vi "Multi-Carrier Modulation Non-Reentrant.vi"(7 "QAM Comparison":enum16{"MT Modulate", "Homebrew"}(ring), 8 "DataLen":i32=512, 9 "QAM Complexity":T1(ring), 10 "Number of Subcarriers":i32, 11 "Lowest f":dbl=1.0 format="%0.2p") -> (0 "FFT Complex":cluster{"f0":dbl, "df":dbl, "real part":dbl[]}(graph), 1 "FFT Real":cluster{"f0":dbl, "df":dbl, "real part":dbl[]}(graph), 2 "output waveform":waveform(cdb), 3 "Waveform Chart":dbl[][](graph))   [LabVIEW 2018]
uses:
  <vilib>/Analysis/Matrix/Datatypes/ComplexMatrix.ctl
  <vilib>/Analysis/Matrix/Numeric/Conversions/Matrix To Array - CM.vi
  <vilib>/measure/maspectr.llb/FFT Spectrum (Real-Im) for 1 Chan.vi
  <vilib>/measure/NI_MAPro.lvlib
  <vilib>/Analysis/Matrix/NI_Matrix.lvlib
panel:
  out "Minimum Sampling Rate":dbl
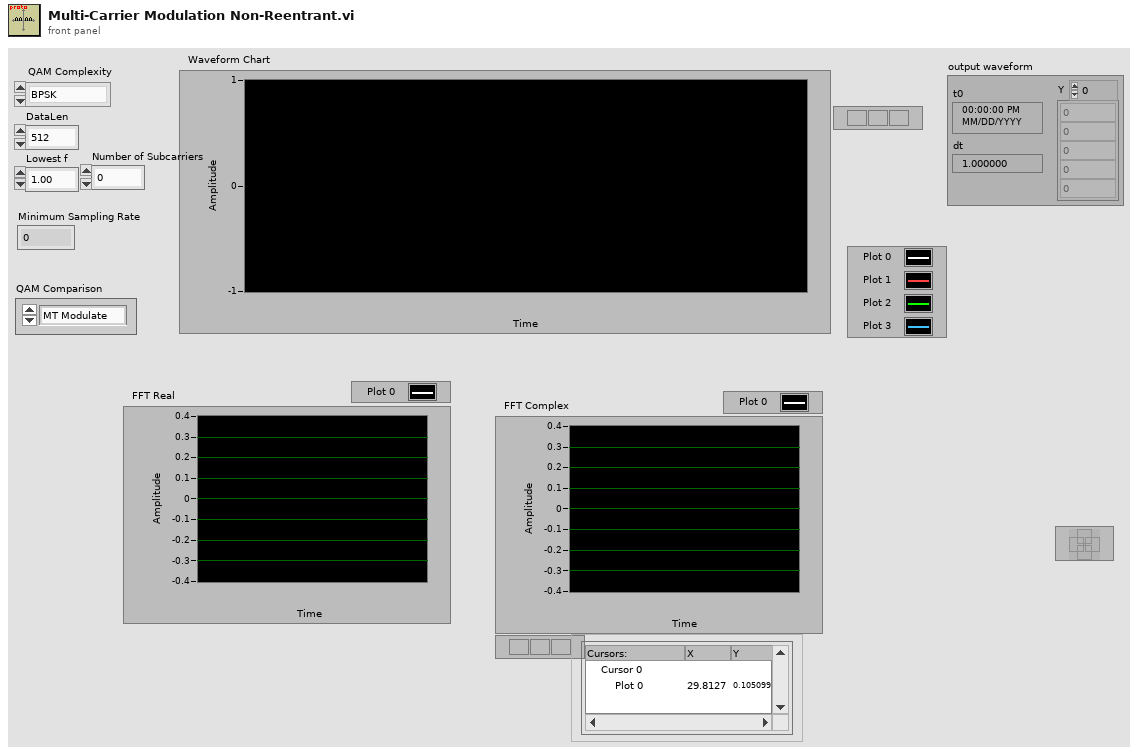
[diagram p1: front panel]
types:
  T1 = enum16{"BPSK", "QPSK", "16-QAM", "64-QAM", "256-QAM"}
  T2 = typedef "NI_Matrix.lvlib/ComplexMatrix.ctl" = cdb[][]
  T3 = cluster{"f0":dbl, "df":dbl, "imaginary part":dbl[]}
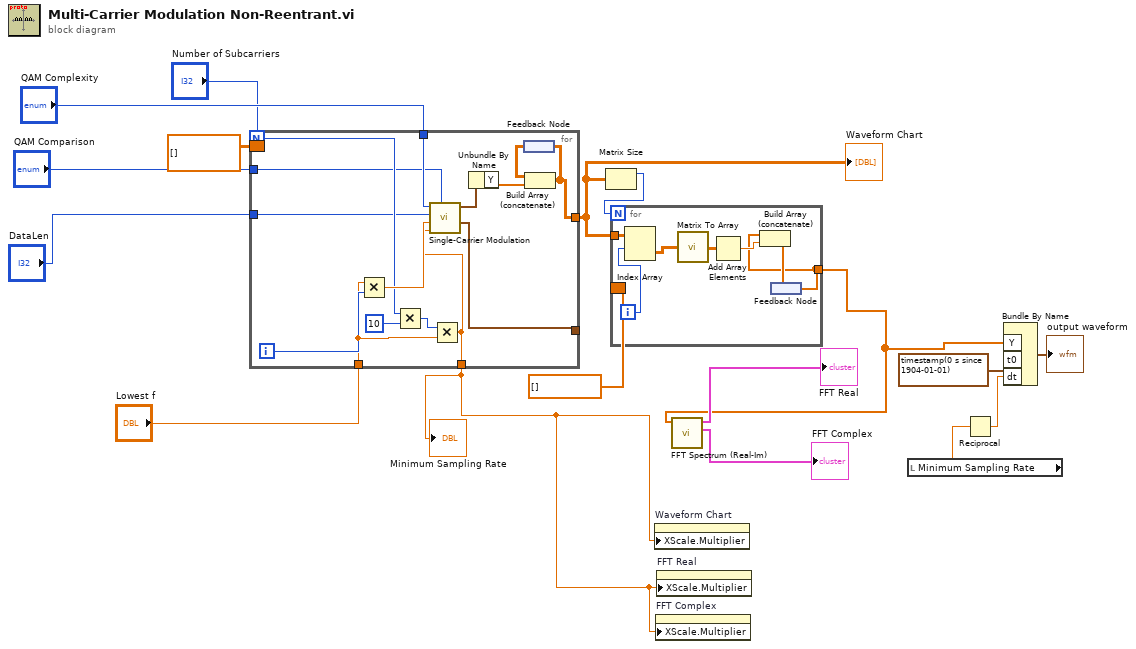
[diagram p0: block diagram]
diagram:
  n1 = for {
    N: "Number of Subcarriers" -> [w30]
    tunnel: "Lowest f" -> [w23]
    tunnel: "DataLen" -> [w28]
    tunnel: "QAM Complexity" -> [w27]
    tunnel: "QAM Comparison" -> [w26]
    tunnel: [w25] -> _
    tunnel: [w19] -> w10
    border: T2 [] ("Complex Matrix") -> [_]
    tunnel: [w18] -> w3
    i -> [w32]
    n2 = Multiply(x=w23, y=w32) -> (x*y=w31:dbl)
    n3 = Multiply(x=w30, y=10) -> (x*y=w24:i32)
    n4 = Multiply(x=w24, y=w23) -> (x*y=w18:dbl)
    n5 = call "Single-Carrier Modulation.vi"("QAM Comparison"=w26, "Sampling Rate"=w18, "frequency"=w31, "DataLen"=w28, "QAM Complexity"=w27) -> ("sampling info"=w25:cluster{"Fs":dbl, "#s":dbl}, "waveform"=w22:waveform(cdb))  [unwired: 5 in]
    n6 = Unbundle By Name(w22) -> ("Y"=w21:cdb[])
    n7 = feedback #1() -> (w20:T2)
    n8 = Build Array (concatenate)(w20, w21) -> (w19:T2)
    n9 = feedback-in #1(w19) -> ()
  }
  "Minimum Sampling Rate" <- w3
  "Waveform Chart" <- w10
  n10 = Matrix Size(0:w10) -> (1:w8:i32)  [unwired: 1 out]
  n11 = for {
    N: w8 -> [_]
    tunnel: w10 -> [w34]
    tunnel: [w35] -> w6
    border: cdb[] [] -> [_]
    i -> [w33]
    n12 = Index Array(array=w34, index (row)=w33) -> (element=w39:T2)  [unwired: 1 in]
    n13 = call-poly <vilib>:"Matrix To Array.vi"("Complex Matrix"=w39) -> ("Complex 2D Array"=w38:cdb[][])
    n14 = Add Array Elements(numeric array=w38) -> (sum=w37:cdb)
    n15 = feedback #2() -> (w35:cdb[])
    n16 = Build Array (concatenate)(w35, w37) -> (w36:cdb[])
    n17 = feedback-in #2(w36) -> ()
  }
  n18 = property on="Waveform Chart" class="WFChart (strict)"("XScale.Multiplier"=w3) -> ()  [unwired: 2 in, 2 out]
  n19 = property on="FFT Complex" class="WFGraph (strict)"("XScale.Multiplier"=w3) -> ()  [unwired: 2 in, 2 out]
  n20 = property on="FFT Real" class="WFGraph (strict)"("XScale.Multiplier"=w3) -> ()  [unwired: 2 in, 2 out]
  n21 = call-poly <vilib>:"FFT Spectrum (Real-Im).vi"("time signal"=w6) -> ("imaginary part"=→"FFT Complex":T3, "real part"=→"FFT Real":cluster{"f0":dbl, "df":dbl, "real part":dbl[]})  [unwired: 6 in, 3 out]
  n22 = local read "Minimum Sampling Rate"() -> (w2:dbl)
  n23 = Reciprocal(x=w2) -> (1/x=w4:dbl)
  n24 = Bundle By Name("Y"=w6, "t0"=timestamp(0 s since 1904-01-01), "dt"=w4) -> (→"output waveform":waveform(cdb))  [unwired: 1 in]
